vi "Scan Variant from String__ogtk.vi"(7 "Format String (optional)":string, 8 "Default Value":variant, 9 "error in (no error)":errorcluster, 10 "Initial Scan Location":u32, 11 "Input String":string) -> (0 "Output":variant, 1 "error out":errorcluster, 2 "Offset Past Scan":u32, 3 "Remaining String":string)   [LabVIEW 2009]
panel:
  # "[OpenG VI Tags] ***Do Not Remove***"
  # "Scan Variant From String.vi\n\nOvercomes a limitation of \"Scan From String\" by allowing variant data types to be used/returned. This VI supports variant data for all LabVIEW data types supported by\n\"Scan From String\".  The \"format string\" input may optionally be passed as an variant attribute named \"Format String\"\n\nPlease visit http://www.OpenG.org to learn about the\nOpen Source LabVIEW software movement.\n\nNOTICE -- YOU MUST LEAVE THIS NOTICE IN PLACE.  PER THE TERMS OF THE LICENSE BELOW, YOU MAY SUBLICENSE THIS SOFTWARE \nIN ANY WAY THAT DOES NOT CONFLICT WITH THIS LICENSE.\n\n### BSD License (http://www.opensource.org/licenses/bsd-license.php) Begin ###\n \nCopyright (c) 2002-2004, Jim Kring <jim@jimkring.com>\nCopyright (c) 2004, Michael C. Ashe <michael.ashe@imaginatics.com>\n\nAll rights reserved.\n\nRedistribution and use in source and binary forms, with or without modification, are permitted provided that the following conditions are met:\n\n    * Redistributions of source code must retain the above copyright notice, this list of conditions and the following disclaimer.\n    * Redistributions in binary form must reproduce the above copyright notice, this list of conditions and the following disclaimer in the \n       documentation and/or other materials provided with the distribution.\n    * Neither the name of SciWare, James Kring, Inc., nor the names of its contributors may be used to endorse or promote products derived \n       from this software without specific prior written permission.\n\nTHIS SOFTWARE IS PROVIDED BY THE COPYRIGHT HOLDERS AND CONTRIBUTORS \"AS IS\" AND ANY EXPRESS OR IMPLIED WARRANTIES, \nINCLUDING, BUT NOT LIMITED TO, THE IMPLIED WARRANTIES OF MERCHANTABILITY AND FITNESS FOR A PARTICULAR PURPOSE ARE \nDISCLAIMED. IN NO EVENT SHALL THE COPYRIGHT OWNER OR CONTRIBUTORS BE LIABLE FOR ANY DIRECT, INDIRECT, INCIDENTAL,\n SPECIAL, EXEMPLARY, OR CONSEQUENTIAL DAMAGES (INCLUDING, BUT NOT LIMITED TO, PROCUREMENT OF SUBSTITUTE GOODS OR \nSERVICES; LOSS OF USE, DATA, OR PROFITS; OR BUSINESS INTERRUPTION) HOWEVER CAUSED AND ON ANY THEORY OF LIABILITY, \nWHETHER IN CONTRACT, STRICT LIABILITY, OR TORT (INCLUDING NEGLIGENCE OR OTHERWISE) ARISING IN ANY WAY OUT OF THE USE \nOF THIS SOFTWARE, EVEN IF ADVISED OF THE POSSIBILITY OF SUCH DAMAGE.\n\n### BSD License End ###"
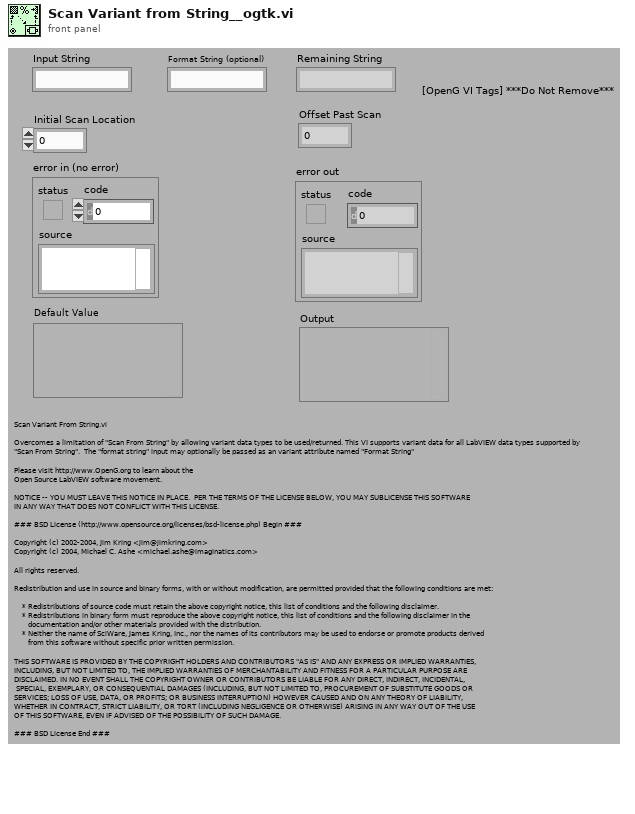
[diagram p1: front panel]
types:
  T1 = typedef "Type Descriptor Enumeration__ogtk.ctl" = enum8{"<Null>", "I8", "I16", "I32", "I64", "U8", "U16", "U32", "U64", "SGL", "DBL", "EXT", "CSG", "CDB", "CXT", "0x0F", "0x10", "0x11", "0x12", "0x13", "0x14", "Enum U8", "Enum U16", "Enum U32", "Enum U64", "SGL PQ", "DBL PQ", "EXT PQ", "CSG PQ", "CDB PQ", "CXT PQ", "0x1F", "0x20", "Boolean", "0x22", "0x23", "0x24", "0x25", "0x26", "0x27", "0x28", "0x29", "0x2A", "0x2B", "0x2C", "0x2D", "0x2E", "0x2F", "String", "0x31", "Path", "Pict", "0x34", "0x35", "0x36", "DAQ", "0x38", "0x39", "0x3A", "0x3B", "0x3C", "0x3D", "0x3E", "0x3F", "Array", "0x41", "0x42", "0x43", "0x44", "0x45", "0x46", "0x47", "0x48", "0x49", "0x4A", "0x4B", "0x4C", "0x4D", "0x4E", "0x4F", "Cluster", "0x51", "0x52", "Variant", "Waveform", "0x55", "0x56", "0x57", "0x58", "0x59", "0x5A", "0x5B", "0x5C", "0x5D", "0x5E", "0x5F", "0x60", "0x61", "0x62", "0x63", "0x64", "0x65", "0x66", "0x67", "0x68", "0x69", "0x6A", "0x6B", "0x6C", "0x6D", "0x6E", "0x6F", "Refnum"}
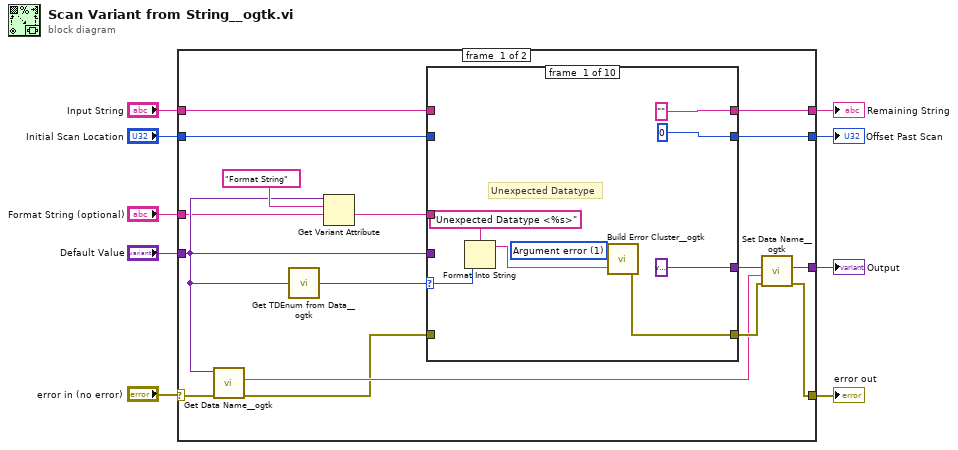
[diagram p0: block diagram]
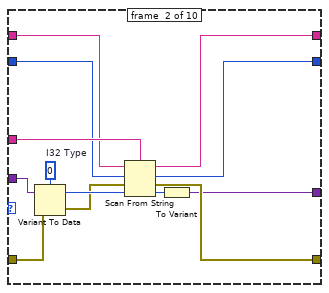
[diagram p2: hidden frame]
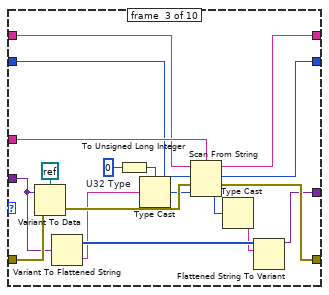
[diagram p3: hidden frame]
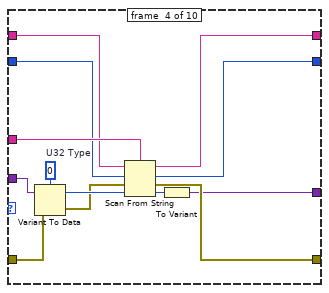
[diagram p4: hidden frame]
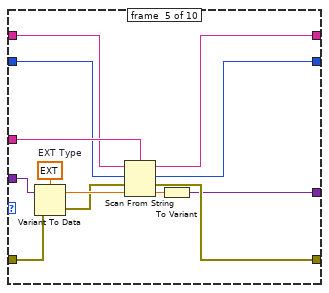
[diagram p5: hidden frame]
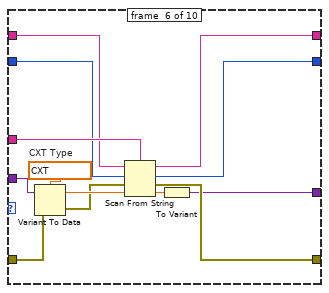
[diagram p6: hidden frame]
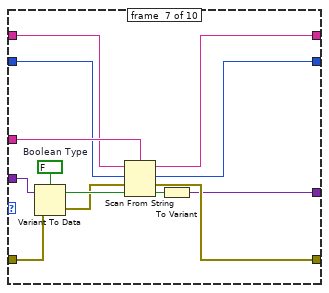
[diagram p7: hidden frame]
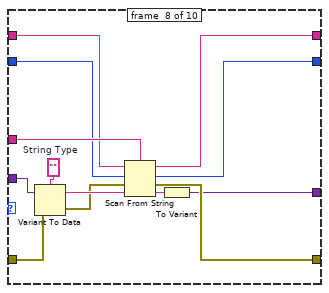
[diagram p8: hidden frame]
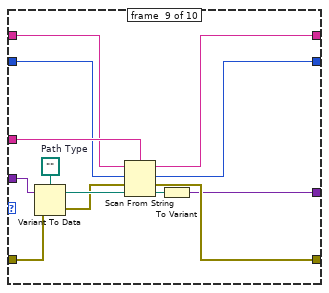
[diagram p9: hidden frame]
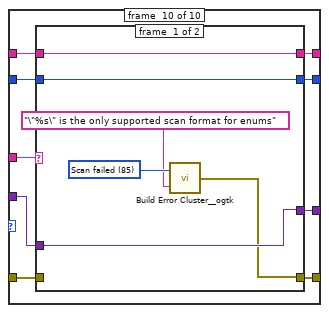
[diagram p10: hidden frame]
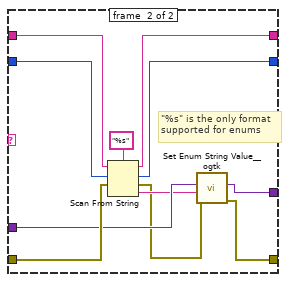
[diagram p11: hidden frame]
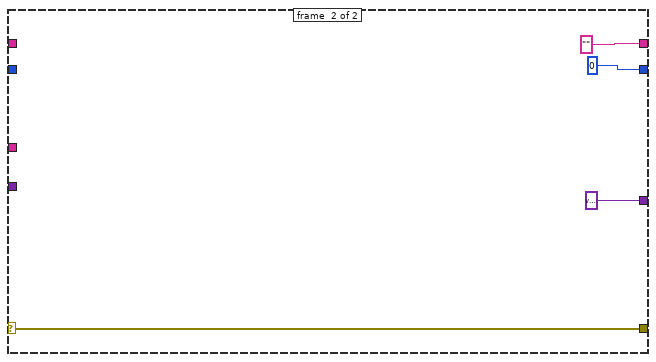
[diagram p12: hidden frame]
diagram:
  n1 = case shown="No Error" "error in (no error)" {
    selector: "error in (no error)" -> [w10 w172]
    tunnel: "Input String" -> [w24 _]
    tunnel: [w23 ""] -> w8
    tunnel: "Format String (optional)" -> [w14 _]
    tunnel: "Default Value" -> [w15 _]
    tunnel: [w18 w172] -> w4
    tunnel: "Initial Scan Location" -> [w22 _]
    tunnel: [w21 u32 0] -> w2
    tunnel: [w19 variant] -> w1
    frame #0 {
      n2 = call <userlib>:"Get Data Name__ogtk.vi"("error in (no error)"=w10, "Data"=w15) -> ("error out"=w11:errorcluster, "Data Name"=w16:string)  [unwired: 7 in, 1 out]
      n3 = call <userlib>:"Get TDEnum from Data__ogtk.vi"("Data"=w15) -> ("Type Descriptor Enumeration"=w12:T1)  [unwired: 4 in]
      n4 = Get Variant Attribute(Variant=w15, name="Format String", default value (empty Variant)=w14) -> (value=w13:string)  [unwired: 1 in, 3 out]
      n5 = case shown="\"Refnum\"" w12 {
        selector: w12 -> [w29 _ _ _ _ _ _ _ _ _]
        tunnel: w15 -> [_ w45 w51 w76 w89 w102 w115 w128 w141 w146]
        tunnel: w13 -> [_ w44 w63 w75 w88 w101 w114 w127 w140 w143]
        tunnel: [w28 w39 w59 w70 w83 w96 w109 w122 w135 w144] -> w17
        tunnel: w11 -> [_ w43 w62 w74 w87 w100 w113 w126 w139 w151]
        tunnel: w24 -> [_ w41 w61 w72 w85 w98 w111 w124 w137 w149]
        tunnel: ["" w40 w60 w71 w84 w97 w110 w123 w136 w148] -> w23
        tunnel: w22 -> [_ w37 w57 w68 w81 w94 w107 w120 w133 w150]
        tunnel: [u32 0 w36 w56 w67 w80 w93 w106 w119 w132 w147] -> w21
        tunnel: [variant w34 w47 w65 w78 w91 w104 w117 w130 w145] -> w20
        frame #0 {
          w30 = 1 items=["No error", "Argument error", "Memory is full", "Out of zone", "End of file", "File already open", "Generic file I/O error", "File not found", "File permission error", "Disk is full", "Duplicate path", "Too many files open", "System feature not enabled", "Resource file not found", "Cannot add resource", "Resource not found", "Image not found", "Image memory error", "Pen does not exist", "Config type invalid", "Config token not found", "Config parse error", "Config memory error", "Bad external code format", "Bad external code offset", "External code not present", "Null window", "Destroy window error", "Null menu", "Print aborted", "Bad print record", "Print driver error", "Windows error during printing", "Memory error during printing", "Print dialog error", "Generic print error", "Invalid device refnum", "Device not found", "Device parameter error", "Device unit error", "Cannot open device", "Device call aborted", "Generic error", "Cancelled by user", "Object ID too low", "Object ID too high", "Object not in heap", "Unknown heap", "Unknown object (invalid DefProc)", "Unknown object (DefProc not in table)", "Message out of range", "Invalid (null) method", "Unknown message", "Manager call not supported", "Bad address", "Network operation in progress", "Network operation timed out", "Connection is busy", "Network attribute not supported", "Network error", "Address in use", "System out of memory", "Connection aborted", "Connection refused", "Not connected", "Already connected", "Connection closed", "Initialization error (interapplication manager)", "Bad occurrence", "Wait on unbound occurrence handler", "Occurrence queue overflow", "Datalog type conflict", "Unused", "Unrecognized type (interapplication manager)", "Memory corrupt", "Failed to make temporary DLL", "Old CIN version", "Drag socket not found", "Failed to load drop-object", "Failed to register OLE object", "Failed to release OLE object", "Format specifier type mismatch", "Unknown format specifier", "Too few format specifiers", "Too many format specifiers", "Scan failed", "Newer CIN version", "Error converting to variant", "Runtime menu error", "Password tampered", "Variant attribute not found", "Incompatible variant data type", "Event data is not available", "Event Store is not present", "Occurrence is not found", "Event Queue is not created", "Event info is not available", "Refnum passed is NULL", "Error retrieving Class GUID", "Error retrieving CoClass GUID", "Error retrieving TypeLib GUID.", "Bad built application magic bytes.", "Specific driver is different from the specific driver associated with the Logical Name.", "There is no session opened to the class driver.", "Max Error", "MAX - Error with config objects", "MAX - Error loading configuration", "MAX - Group not supported"]
          # "Unexpected Datatype"
          n6 = Format Into String(format string="Unexpected Datatype <%s>" ("Format String"), w29) -> (resulting string=w32:string)  [unwired: 2 in, 1 out]
          n7 = call <userlib>:"Build Error Cluster__ogtk.vi"("String to Prepend to source (\"\")"=w32, "code"=w30) -> ("error out"=w28:errorcluster)
        }
        frame #1 {
          w46 = 0  # I32 Type
          n8 = Variant To Data(error in=w43, Variant=w45, type=w46) -> (error out=w38:errorcluster, data=w42:i32)
          n9 = Scan From String(format string=w44, input string=w41, initial scan location=w37, error in=w38, default 1=w42) -> (remaining string=w40:string, offset past scan=w36:u32, error out=w39:errorcluster, output 1=w35:i32)
          n10 = To Variant(anything=w35) -> (Variant=w34:variant)
        }
        frame #2 {
          w53 = u32 0  # U32 Type
          n11 = Variant To Data(error in=w62, Variant=w51, type=refnum<k0> refnum) -> (error out=w58:errorcluster)  [unwired: 1 out]
          n12 = Variant To Flattened String(Variant=w51) -> (data string=w49:string, 1:w50:i16[])
          n13 = To Unsigned Long Integer(number=w53) -> (unsigned 32bit integer=w52:u32)
          n14 = Type Cast(type=w52, x=w49) -> (*(type *) &x=w54:u32)
          n15 = Scan From String(format string=w63, input string=w61, initial scan location=w57, error in=w58, default 1=w54) -> (remaining string=w60:string, offset past scan=w56:u32, error out=w59:errorcluster, output 1=w55:u32)
          n16 = Type Cast(x=w55) -> (*(type *) &x=w48:string)  [unwired: 1 in]
          n17 = Flattened String To Variant(6:w48, 7:w50) -> (3:w47:variant)  [unwired: 1 in, 1 out]
        }
        frame #3 {
          w77 = u32 0  # U32 Type
          n18 = Variant To Data(error in=w74, Variant=w76, type=w77) -> (error out=w69:errorcluster, data=w73:u32)
          n19 = Scan From String(format string=w75, input string=w72, initial scan location=w68, error in=w69, default 1=w73) -> (remaining string=w71:string, offset past scan=w67:u32, error out=w70:errorcluster, output 1=w66:u32)
          n20 = To Variant(anything=w66) -> (Variant=w65:variant)
        }
        frame #4 {
          w90 = ext 0.0  # EXT Type
          n21 = Variant To Data(error in=w87, Variant=w89, type=w90) -> (error out=w82:errorcluster, data=w86:ext)
          n22 = Scan From String(format string=w88, input string=w85, initial scan location=w81, error in=w82, default 1=w86) -> (remaining string=w84:string, offset past scan=w80:u32, error out=w83:errorcluster, output 1=w79:ext)
          n23 = To Variant(anything=w79) -> (Variant=w78:variant)
        }
        frame #5 {
          w103 = cxt 0.0+0.0i  # CXT Type
          n24 = Variant To Data(error in=w100, Variant=w102, type=w103) -> (error out=w95:errorcluster, data=w99:cxt)
          n25 = Scan From String(format string=w101, input string=w98, initial scan location=w94, error in=w95, default 1=w99) -> (remaining string=w97:string, offset past scan=w93:u32, error out=w96:errorcluster, output 1=w92:cxt)
          n26 = To Variant(anything=w92) -> (Variant=w91:variant)
        }
        frame #6 {
          w116 = FALSE  # Boolean Type
          n27 = Variant To Data(error in=w113, Variant=w115, type=w116) -> (error out=w108:errorcluster, data=w112:bool)
          n28 = Scan From String(format string=w114, input string=w111, initial scan location=w107, error in=w108, default 1=w112) -> (remaining string=w110:string, offset past scan=w106:u32, error out=w109:errorcluster, output 1=w105:bool)
          n29 = To Variant(anything=w105) -> (Variant=w104:variant)
        }
        frame #7 {
          w129 = ""  # String Type
          n30 = Variant To Data(error in=w126, Variant=w128, type=w129) -> (error out=w121:errorcluster, data=w125:string)
          n31 = Scan From String(format string=w127, input string=w124, initial scan location=w120, error in=w121, default 1=w125) -> (remaining string=w123:string, offset past scan=w119:u32, error out=w122:errorcluster, output 1=w118:string)
          n32 = To Variant(anything=w118) -> (Variant=w117:variant)
        }
        frame #8 {
          w142 = path ""  # Path Type
          n33 = Variant To Data(error in=w139, Variant=w141, type=w142) -> (error out=w134:errorcluster, data=w138:path)
          n34 = Scan From String(format string=w140, input string=w137, initial scan location=w133, error in=w134, default 1=w138) -> (remaining string=w136:string, offset past scan=w132:u32, error out=w135:errorcluster, output 1=w131:path)
          n35 = To Variant(anything=w131) -> (Variant=w130:variant)
        }
        frame #9 {
          n36 = case shown="\"\", \"%s\"" w143 {
            tunnel: w151 -> [_ w168]
            tunnel: w150 -> [w156 w167]
            tunnel: w149 -> [w157 w166]
            tunnel: [w157 w165] -> w148
            tunnel: [w156 w164] -> w147
            tunnel: w146 -> [w155 w163]
            tunnel: [w155 w161] -> w145
            tunnel: [w154 w159] -> w144
            frame #0 {
              w153 = 85 items=["No error", "Argument error", "Memory is full", "Out of zone", "End of file", "File already open", "Generic file I/O error", "File not found", "File permission error", "Disk is full", "Duplicate path", "Too many files open", "System feature not enabled", "Resource file not found", "Cannot add resource", "Resource not found", "Image not found", "Image memory error", "Pen does not exist", "Config type invalid", "Config token not found", "Config parse error", "Config memory error", "Bad external code format", "Bad external code offset", "External code not present", "Null window", "Destroy window error", "Null menu", "Print aborted", "Bad print record", "Print driver error", "Windows error during printing", "Memory error during printing", "Print dialog error", "Generic print error", "Invalid device refnum", "Device not found", "Device parameter error", "Device unit error", "Cannot open device", "Device call aborted", "Generic error", "Cancelled by user", "Object ID too low", "Object ID too high", "Object not in heap", "Unknown heap", "Unknown object (invalid DefProc)", "Unknown object (DefProc not in table)", "Message out of range", "Invalid (null) method", "Unknown message", "Manager call not supported", "Bad address", "Network operation in progress", "Network operation timed out", "Connection is busy", "Network attribute not supported", "Network error", "Address in use", "System out of memory", "Connection aborted", "Connection refused", "Not connected", "Already connected", "Connection closed", "Initialization error (interapplication manager)", "Bad occurrence", "Wait on unbound occurrence handler", "Occurrence queue overflow", "Datalog type conflict", "Unused", "Unrecognized type (interapplication manager)", "Memory corrupt", "Failed to make temporary DLL", "Old CIN version", "Drag socket not found", "Failed to load drop-object", "Failed to register OLE object", "Failed to release OLE object", "Format specifier type mismatch", "Unknown format specifier", "Too few format specifiers", "Too many format specifiers", "Scan failed", "Newer CIN version", "Error converting to variant", "Runtime menu error", "Password tampered", "Variant attribute not found", "Incompatible variant data type", "Event data is not available", "Event Store is not present", "Occurrence is not found", "Event Queue is not created", "Event info is not available", "Refnum passed is NULL", "Error retrieving Class GUID", "Error retrieving CoClass GUID", "Error retrieving TypeLib GUID.", "Bad built application magic bytes.", "Specific driver is different from the specific driver associated with the Logical Name.", "There is no session opened to the class driver.", "Max Error", "MAX - Error with config objects", "MAX - Error loading configuration", "MAX - Group not supported"]
              n37 = call <userlib>:"Build Error Cluster__ogtk.vi"("String to Prepend to source (\"\")"="\"%s\" is the only supported scan format for enums" ("String to Prepend to source (\"\")"), "code"=w153) -> ("error out"=w154:errorcluster)
            }
            frame #1 {
              # "\"%s\" is the only format\nsupported for enums"
              n38 = Scan From String(format string="%s" ("Format String"), input string=w166, initial scan location=w167, error in=w168) -> (remaining string=w165:string, offset past scan=w164:u32, error out=w160:errorcluster, output 1=w162:string)  [unwired: 1 in]
              n39 = call <userlib>:"Set Enum String Value__ogtk.vi"("error in (no error)"=w160, "String Value"=w162, "Default Enum Value"=w163) -> ("error out"=w159:errorcluster, "Enum"=w161:variant)  [unwired: 7 in]
            }
          }
        }
      }
      n40 = call <userlib>:"Set Data Name__ogtk.vi"("error in (no error)"=w17, "Data Name"=w16, "Data"=w20) -> ("error out"=w18:errorcluster, "Renamed Data"=w19:variant)  [unwired: 7 in]
    }
    frame #1 {
    }
  }
  "Remaining String" <- w8
  "error out" <- w4
  "Offset Past Scan" <- w2
  "Output" <- w1
